vi "AutoRightDrive.vi"() -> ()   [LabVIEW 2016]
panel:
  in  "Auto Right Drive contr":dbl
  out "Auto Right Drive indic":dbl
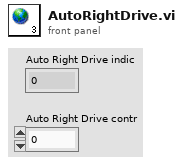
[diagram p1: front panel]
diagram:
